vi "Write Overlay Positions.vi"(8 "error in (no error)":errorcluster, 10 "Overlay Positions":cluster{"x":i16, "y":i16}[](array[cluster]), 11 "Analyze Results Distanz in":refnum<class "Analyze Results Distanz.lvclass">) -> (0 "error out":errorcluster, 3 "Analyze Results Distanz out":refnum<class "Analyze Results Distanz.lvclass">)   [LabVIEW 2014, in "Analyze Results Distanz.lvclass"]
uses:
  Analyze Results Distanz.lvclass
  Analyze Results Distanz.lvclass/Analyze Results Distanz.ctl
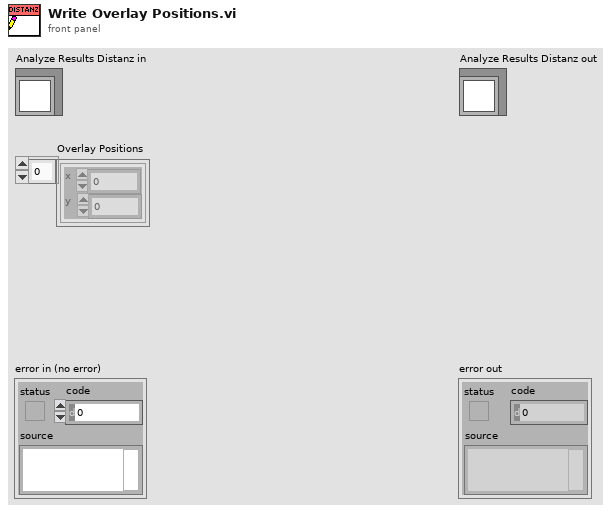
[diagram p1: front panel]
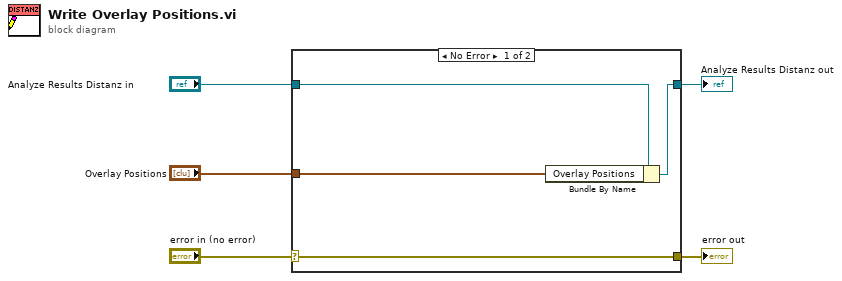
[diagram p0: block diagram]
diagram:
  n1 = case shown="No Error" "error in (no error)" {
    selector: "error in (no error)" -> [w9 w10]
    tunnel: [w9 w10] -> w4
    tunnel: [w7 w11] -> w2
    tunnel: "Analyze Results Distanz in" -> [w8 w11]
    tunnel: "Overlay Positions" -> [w6 _]
    frame No Error {
      n2 = Bundle By Name(cluster=w8, "Overlay Positions"=w6) -> (w7:refnum<class "Analyze Results Distanz.lvclass">)
    }
    frame Error {
    }
  }
  "error out" <- w4
  "Analyze Results Distanz out" <- w2
